vi "Append-FRD.vi"(10 "experiment-data":T2) -> (3 "FRD-out":T1)   [LabVIEW 2017]
uses:
  controls/SS_experimental-data.ctl
  controls/SS_FourierData.ctl
  controls/FrdData.ctl
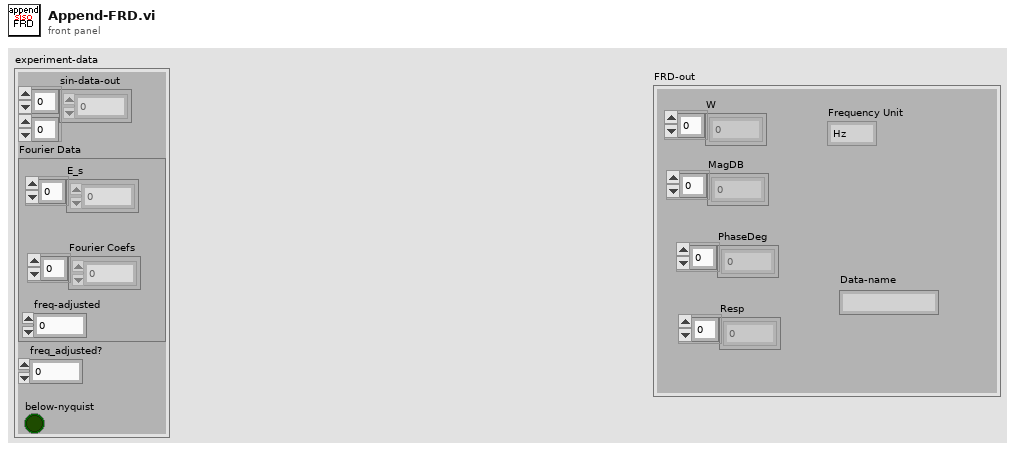
[diagram p1: front panel]
types:
  T1 = typedef "FrdData.ctl" = cluster{"Frequency Unit":enum16{"Hz", "rad/s"}, "W":dbl[], "MagDB":dbl[], "PhaseDeg":dbl[], "Resp":cdb[], "Data-name":string}
  T2 = typedef "SS_experimental-data.ctl" = cluster{"sin-data-out":dbl[][], "Fourier Data":T3, "freq_adjusted?":dbl, "below-nyquist":bool}
  T3 = typedef "SS_FourierData.ctl" = cluster{"E_s":dbl[], "Fourier Coefs":cdb[], "freq-adjusted":dbl}
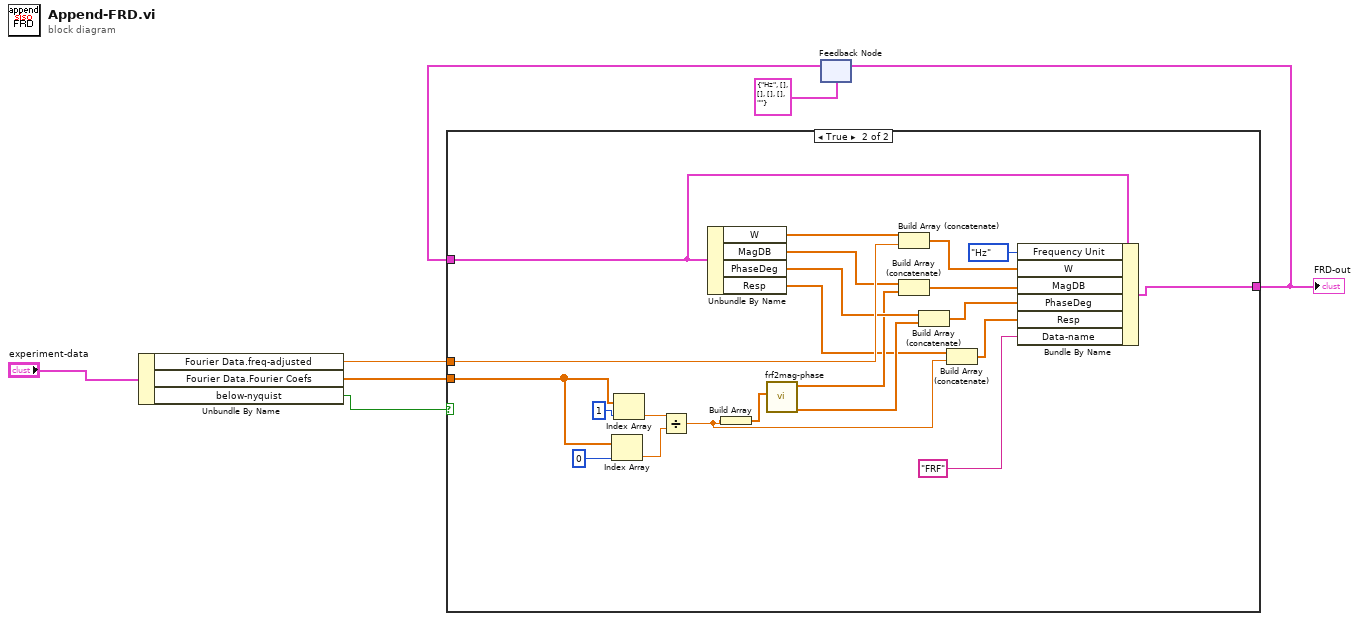
[diagram p0: block diagram]
diagram:
  n1 = Unbundle By Name("experiment-data") -> ("Fourier Data.freq-adjusted"=w5:dbl, "Fourier Data.Fourier Coefs"=w6:cdb[], "below-nyquist"=w4:bool)
  n2 = feedback #1(T1 {"Frequency Unit"=enum."Hz", "W"=[], "MagDB"=[], "PhaseDeg"=[], "Resp"=[], "Data-name"=""} ("FRD-in")) -> (w2:T1)
  n3 = case shown="True" w4 {
    tunnel: w6 -> [_ w27]
    tunnel: w5 -> [_ w23]
    tunnel: [w8 w15] -> w3
    tunnel: w2 -> [w8 w9]
    frame False {
    }
    frame True {
      n4 = Index Array(array=w27, index=0) -> (element=w30:cdb)
      n5 = Index Array(array=w27, index=1) -> (element=w26:cdb)
      n6 = Divide(x=w26, y=w30) -> (x/y=w14:cdb)
      n7 = Unbundle By Name(w9) -> ("W"=w24:dbl[], "MagDB"=w21:dbl[], "PhaseDeg"=w18:dbl[], "Resp"=w12:cdb[])
      n8 = Build Array(w14) -> (w25:cdb[])
      n9 = call "frf2mag-phase.vi"("G_frf"=w25) -> ("phase [deg]"=w16:dbl[], "mag-dB"=w17:dbl[])  [unwired: 9 in]
      n10 = Build Array (concatenate)(w24, w23) -> (w22:dbl[])
      n11 = Build Array (concatenate)(w21, w17) -> (w20:dbl[])
      n12 = Build Array (concatenate)(w18, w16) -> (w19:dbl[])
      n13 = Build Array (concatenate)(w12, w14) -> (w13:cdb[])
      n14 = Bundle By Name(cluster=w9, "Frequency Unit"=enum16{"Hz", "rad/s"}."Hz", "W"=w22, "MagDB"=w20, "PhaseDeg"=w19, "Resp"=w13, "Data-name"="FRF") -> (w15:T1)
    }
  }
  "FRD-out" <- w3
  n15 = feedback-in #1(w3) -> ()
